vi "Uppercase.vi"() -> ()   [LabVIEW 2016]
panel:
  in  "String":string
  in  "stop":bool
  # "Character to Caps while typing during runtime"
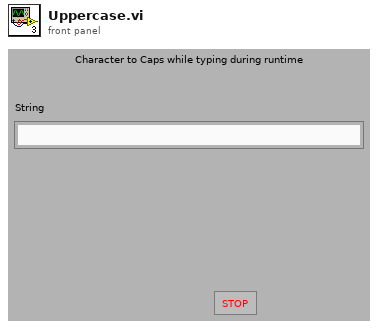
[diagram p1: front panel]
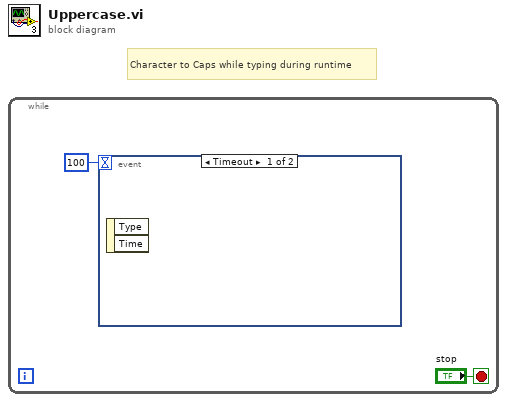
[diagram p0: block diagram]
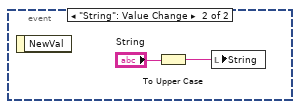
[diagram p2: hidden frame]
diagram:
  # "Character to Caps while typing during runtime"
  n1 = while {
    stop <- "stop" stop-if-true
    n2 = event shown="[0] Timeout" {
      selector: _ -> [_ _]
      dyn-events: _ -> [_ _]
      timeout: 100 -> [_ _]
      event Timeout {
        n3 = event-data() -> ()  [unwired: 1 in, 2 out]
      }
      event "String": Value Change {
        n4 = event-data() -> ()  [unwired: 1 in, 1 out]
        n5 = To Upper Case(1:"String") -> (0:w3:string)
        n6 = local write "String"(w3) -> ()
      }
    }
  }
